vi "Create Stop Event.vi"(8 "error in (no error)":errorcluster) -> (0 "error out":errorcluster, 3 "Stop Event out":refnum<user-event>)   [LabVIEW 2016, in "Trace Grabber.lvlib"]
uses:
  Trace Grabber.lvlib
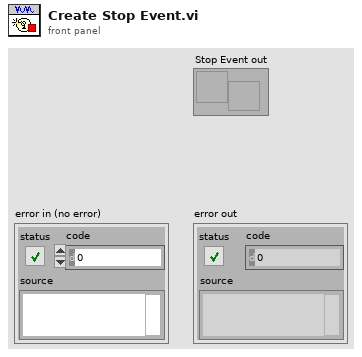
[diagram p1: front panel]
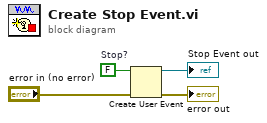
[diagram p0: block diagram]
diagram:
  w2 = FALSE  # Stop?
  n1 = Create User Event(user event datatype=w2, error in="error in (no error)") -> (user event=→"Stop Event out":refnum<user-event>, error out=→"error out":errorcluster)
